vi "Bottle_assignments.vi"(1 "Odour bottles":T2(array[cluster])=[[{"Mixture components"=[{"Name"="MINERAL OIL", "CID"=0, "Volatility"=0.0}], "Name"="B1 (Bl)", "VPs"="0.0E+0", "Proportion"=[{"Numeric"=100.0}], "Selected"=FALSE, "Counter"=TRUE}, {"Mixture components"=[{"Name"="Methyl benzoate", "CID"=8103, "Volatility"=0.38}, {"Name"="Menthone", "CID"=8063, "Volatility"=0.28}], "Name"="B3 (ME2)", "VPs"="3.3E-1 ± 21%", "Proportion"=[{"Numeric"=50.0}, {"Numeric"=50.0}], "Selected"=TRUE, "Counter"=FALSE}, {"Mixture components"=[{"Name"="Decanol", "CID"=460, "Volatility"=0.00851}], "Name"="B5 (C4f)", "VPs"="8.5E-3", "Proportion"=[{"Numeric"=100.0}], "Selected"=FALSE, "Counter"=FALSE}, {"Mixture components"=[{"Name"="Acetophenone", "CID"=8174, "Volatility"=0.45}, {"Name"="Fenchone", "CID"=8635, "Volatility"=0.82}], "Name"="B7 (ME1)", "VPs"="6.4E-1 ± 41%", "Proportion"=[{"Numeric"=50.0}, {"Numeric"=50.0}], "Selected"=FALSE, "Counter"=FALSE}], [{"Mixture components"=[{"Name"="MINERAL OIL", "CID"=0, "Volatility"=0.0}], "Name"="B2 (Bl)", "VPs"="0.0E+0", "Proportion"=[{"Numeric"=100.0}], "Selected"=FALSE, "Counter"=TRUE}, {"Mixture components"=[{"Name"="Octanol", "CID"=7439, "Volatility"=0.0794}], "Name"="B4 (C4cA)", "VPs"="7.9E-2", "Proportion"=[{"Numeric"=100.0}], "Selected"=FALSE, "Counter"=FALSE}, {"Mixture components"=[{"Name"="MINERAL OIL", "CID"=0, "Volatility"=0.0}], "Name"="B6 (Bl)", "VPs"="0.0E+0", "Proportion"=[{"Numeric"=100.0}], "Selected"=FALSE, "Counter"=FALSE}, {"Mixture components"=[{"Name"="Heptanoic acid ", "CID"=957, "Volatility"=0.0107}], "Name"="B8 (C3cA)", "VPs"="1.1E-2", "Proportion"=[{"Numeric"=100.0}], "Selected"=FALSE, "Counter"=FALSE}], [{"Mixture components"=[{"Name"="MINERAL OIL", "CID"=0, "Volatility"=0.0}], "Name"="B9 (Bl)", "VPs"="0.0E+0", "Proportion"=[{"Numeric"=100.0}], "Selected"=FALSE, "Counter"=TRUE}, {"Mixture components"=[{"Name"="Geranyl acetate", "CID"=6985, "Volatility"=0.03}, {"Name"="Dimethylacetophenone", "CID"=7144, "Volatility"=0.063}], "Name"="B11 (MW1)", "VPs"="4.6E-2 ± 50%", "Proportion"=[{"Numeric"=50.0}, {"Numeric"=50.0}], "Selected"=FALSE, "Counter"=FALSE}, {"Mixture components"=[{"Name"="Geraniol", "CID"=6405, "Volatility"=0.03}, {"Name"="Phenyl butanone", "CID"=7762, "Volatility"=0.1}], "Name"="B13 (MW2)", "VPs"="6.5E-2 ± 76%", "Proportion"=[{"Numeric"=50.0}, {"Numeric"=50.0}], "Selected"=FALSE, "Counter"=FALSE}, {"Mixture components"=[{"Name"="Methylheptanoic acid", "CID"=1032, "Volatility"=0.018}], "Name"="B15 (C3f)", "VPs"="1.8E-2", "Proportion"=[{"Numeric"=100.0}], "Selected"=FALSE, "Counter"=FALSE}], [{"Mixture components"=[{"Name"="MINERAL OIL", "CID"=0, "Volatility"=0.0}], "Name"="B10 (Bl)", "VPs"="0.0E+0", "Proportion"=[{"Numeric"=100.0}], "Selected"=FALSE, "Counter"=FALSE}, {"Mixture components"=[{"Name"="Valeric acid", "CID"=8025, "Volatility"=0.196}], "Name"="B12 (C3cB)", "VPs"="2.0E-1", "Proportion"=[{"Numeric"=100.0}], "Selected"=FALSE, "Counter"=FALSE}, {"Mixture components"=[{"Name"="Nonanol", "CID"=4133, "Volatility"=0.0227}], "Name"="B14 (C4cB)", "VPs"="2.3E-2", "Proportion"=[{"Numeric"=100.0}], "Selected"=FALSE, "Counter"=FALSE}, {"Mixture components"=[{"Name"="Hydroxacetophenone", "CID"=7462, "Volatility"=0.0856}], "Name"="B16 (Ol)", "VPs"="8.6E-2", "Proportion"=[{"Numeric"=100.0}], "Selected"=FALSE, "Counter"=FALSE}]], 2 "Active bottles":i32[](array[numeric])) -> (0 "Bottle assignments":T1)   [LabVIEW 2016]
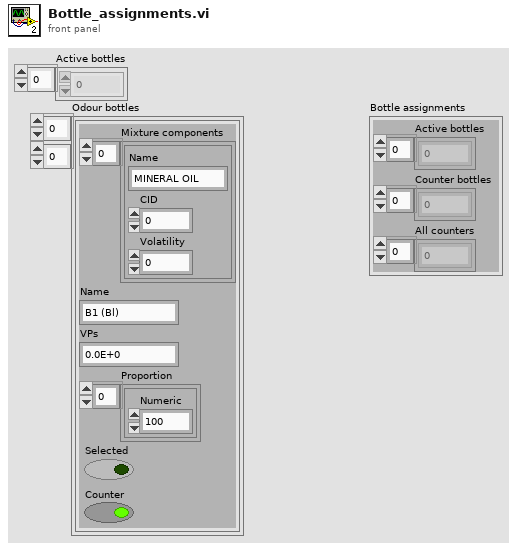
[diagram p1: front panel]
types:
  T1 = cluster{"Active bottles":i32[], "Counter bottles":i32[], "All counters":i32[]}
  T2 = cluster{"Mixture components":cluster{"Name":string, "CID":i32, "Volatility":dbl}[], "Name":string, "VPs":string, "Proportion":cluster{"Numeric":dbl}[], "Selected":bool, "Counter":bool}[][]
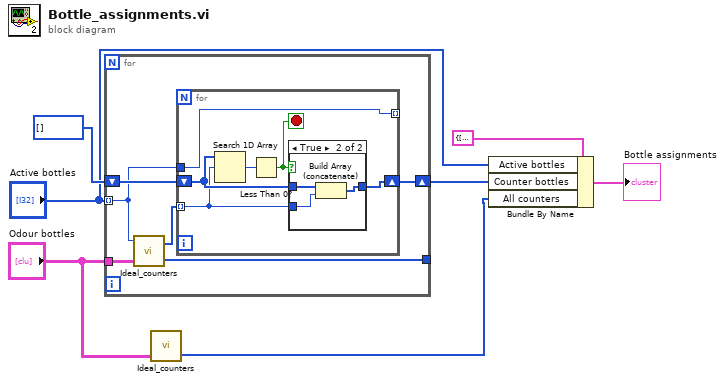
[diagram p0: block diagram]
diagram:
  n1 = for {
    tunnel: "Active bottles" -> [w11] mode=indexing
    shift-right: [w12] -> w5
    shift-left: i32[] [] -> [w13]
    tunnel: "Odour bottles" -> [w10]
    tunnel: [w8] -> _
    n2 = call "Ideal_counters.vi"("Odour bottles"=w10, "Bottle"=w11) -> ("All counters"=w8:i32[], "Ideal counter order"=w9:i32[])  [unwired: 1 in]
    n3 = for {
      shift-right: [w16] -> w12
      shift-left: w13 -> [w17]
      tunnel: [w19] -> _ mode=indexing
      tunnel: w11 -> [w19]
      tunnel: w9 -> [w14] mode=indexing
      stop <- w15 stop-if-true
      n4 = Search 1D Array(1D array=w17, element=w14) -> (index of element=w18:i32)  [unwired: 1 in]
      n5 = Less Than 0?(x=w18) -> (x < 0?=w15:bool)
      n6 = case shown="True" w15 {
        tunnel: w17 -> [w20 w23]
        tunnel: [w20 w22] -> w16
        tunnel: w14 -> [_ w21]
        frame False {
        }
        frame True {
          n7 = Build Array (concatenate)(w23, w21) -> (w22:i32[])
        }
      }
    }
  }
  n8 = call "Ideal_counters.vi"("Odour bottles"="Odour bottles") -> ("All counters"=w1:i32[])  [unwired: 2 in, 1 out]
  n9 = Bundle By Name(cluster=T1 {"Active bottles"=[], "Counter bottles"=[], "All counters"=[0, 1, 8, 9]}, "Active bottles"="Active bottles", "Counter bottles"=w5, "All counters"=w1) -> (→"Bottle assignments":T1)
